vi "AnalyseLV.vi"(8 "error in (no error)":errorcluster, 10 "ImageData":T2, 11 "FluorescenceAnalyser in":refnum<class "FluorescenceAnalyser.lvclass">) -> (0 "error out":errorcluster, 3 "FluorescenceAnalyser out":refnum<class "FluorescenceAnalyser.lvclass">)   [LabVIEW 2009, in "Tools.lvlib" / "Imaging.lvlib" / "FluorescenceAnalyser.lvclass"]
uses:
  FluorescenceAnalyser.lvclass
  <vilib>/Analysis/NI_AALBase.lvlib
  ImageAnalyser.lvclass
panel:
  out "Image":T1(plugin-control)
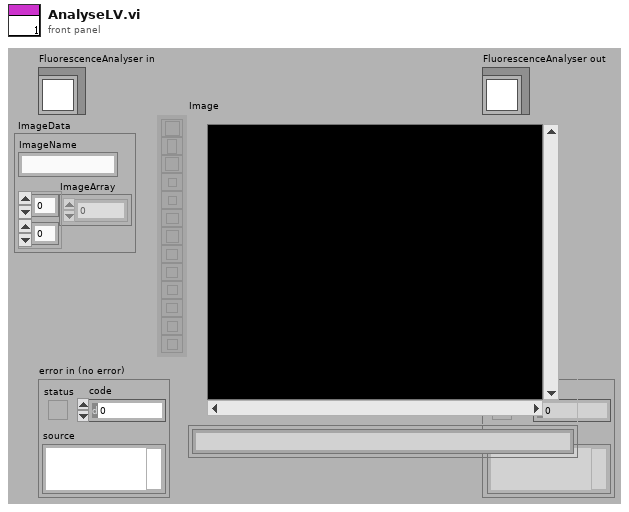
[diagram p1: front panel]
types:
  T1 = typedef "IMAQ Image.ctl" = refnum<image>
  T2 = cluster{"ImageName":string, "ImageArray":sgl[][]}
  T3 = cluster{"Name":string, "Results":dbl[], "AnalysisType":string}
  T4 = cluster{"Objects":u16, "Threshold":i32, "Reject Border":bool, "Fill Holes":bool, "Min Object Size":bool, "Min Size":i32, "Max Object Size":bool, "Max Size":i32, "Show Search Area":bool, "Show Center":bool, "Show Bounding Box":bool}
  T5 = typedef "Image Type" = u32
  T6 = cluster{"Object Center":cluster{"X":sgl, "Y":sgl}, "Bounding Box":cluster{"X Left":i32, "Y Top":i32, "X Right":i32, "Y Bottom":i32}, "Area":sgl, "Orientation":sgl, "Aspect Ratio":sgl, "Nb Holes":i32}[]
  T7 = cluster{"Object Center":cluster{"X":sgl, "Y":sgl}, "Bounding Box":cluster{"X Left":i32, "Y Top":i32, "X Right":i32, "Y Bottom":i32}, "Area":sgl, "Orientation":sgl, "Aspect Ratio":sgl, "Nb Holes":i32}
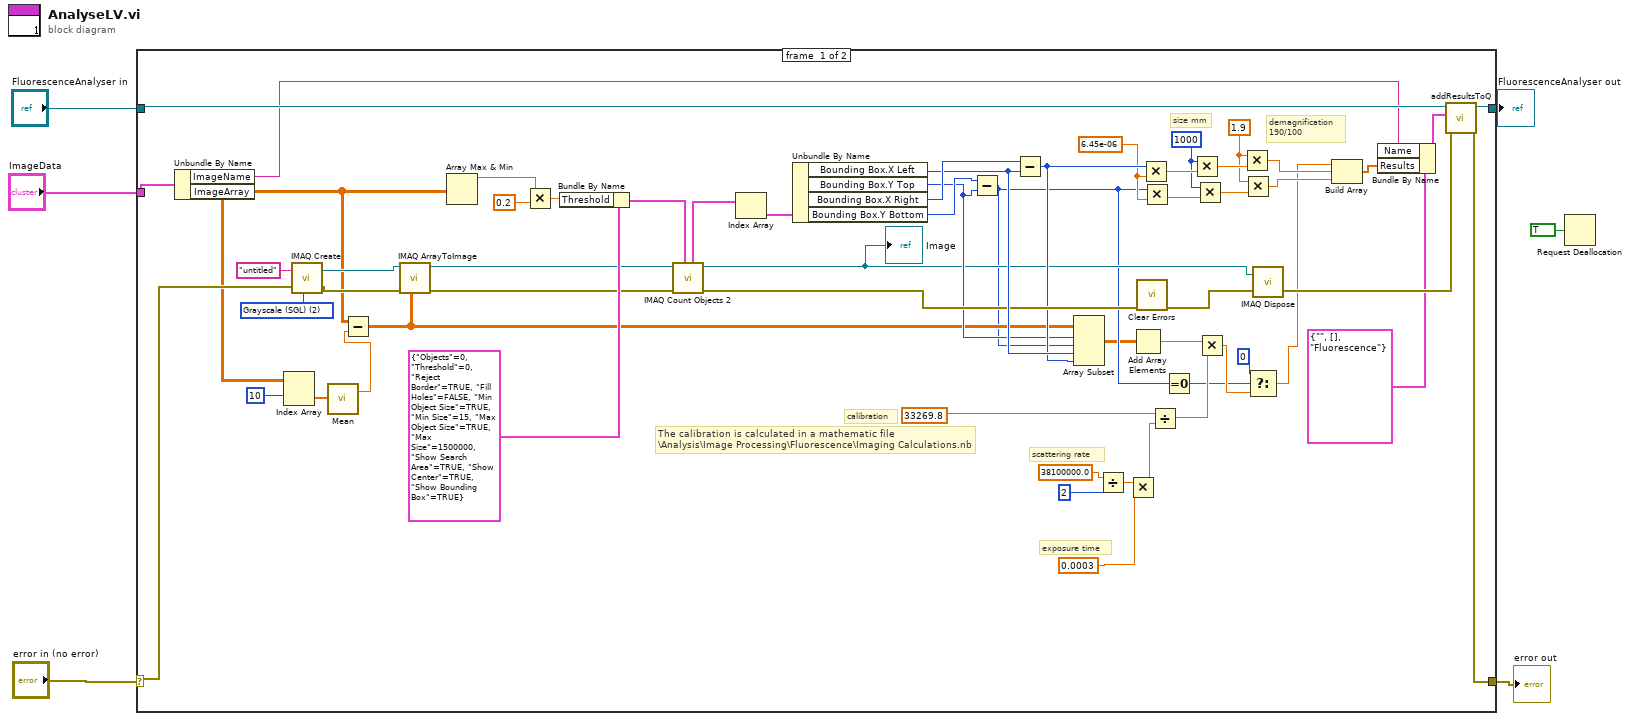
[diagram p0: block diagram]
diagram:
  n1 = case shown="No Error" "error in (no error)" {
    selector: "error in (no error)" -> [w48 w67]
    tunnel: [w33 w67] -> w5
    tunnel: [w35 w66] -> w3
    tunnel: "FluorescenceAnalyser in" -> [w34 w66]
    tunnel: "ImageData" -> [w65 _]
    frame #0 {
      w15 = 1.9
      w28 = 1000
      w46 = 6.45e-06
      w50 = T5 2 items=["Grayscale (U8)", "Grayscale (I16)", "Grayscale (SGL)", "Complex (CSG)", "RGB (U32)", "HSL (U32)", "RGB (U64)", "Grayscale (U16)"] ("Image Type")
      # "The calibration is calculated in a mathematic file\n\\Analysis\\Image Processing\\Fluorescence\\Imaging Calculations.nb"
      # "demagnification\n190/100"
      # "size mm"
      # "exposure time"
      # "scattering rate"
      # "calibration"
      n2 = Unbundle By Name(w65) -> ("ImageName"=w21:string, "ImageArray"=w24:sgl[][])
      n3 = Index Array(array=w24, index (row)=10) -> (element=w42:sgl[])  [unwired: 1 in]
      n4 = call "IMAQ Create"("Image Name"="untitled", "Image Type"=w50, "error in (no error)"=w48) -> ("New Image"=w64:T1, "error out"=w63:errorcluster)  [unwired: 2 in]
      n5 = call <vilib>:"Mean.vi"("X"=w42) -> ("mean"=w10:dbl)  [unwired: 1 out]
      n6 = Subtract(x=w24, y=w10) -> (x-y=w14:dbl[][])
      n7 = call "IMAQ ArrayToImage"("Image Pixels (Float)"=w14, "error in (no error)"=w63, "Image"=w64) -> ("error out"=w55:errorcluster, "Image Out"=w56:T1)  [unwired: 7 in]
      n8 = Array Max & Min(array=w24) -> (max value=w59:sgl)  [unwired: 3 out]
      n9 = Multiply(x=w59, y=0.2) -> (x*y=w60:dbl)
      n10 = Bundle By Name(cluster=T4 {"Objects"=0, "Threshold"=0, "Reject Border"=TRUE, "Fill Holes"=FALSE, "Min Object Size"=TRUE, "Min Size"=15, "Max Object Size"=TRUE, "Max Size"=1500000, "Show Search Area"=TRUE, "Show Center"=TRUE, "Show Bounding Box"=TRUE} ("Settings"), "Threshold"=w60) -> (w57:T4)
      n11 = call "IMAQ Count Objects 2"("Settings"=w57, "error in (no error)"=w55, "Image"=w56) -> ("error out"=w49:errorcluster, "Image Out"=w27:T1, "Objects"=w54:T6)  [unwired: 4 in, 2 out]
      "Image" <- w27
      n12 = Index Array(array=w54) -> (element=w53:T7)  [unwired: 1 in]
      n13 = Unbundle By Name(w53) -> ("Bounding Box.X Left"=w51:i32, "Bounding Box.Y Top"=w31:i32, "Bounding Box.X Right"=w52:i32, "Bounding Box.Y Bottom"=w32:i32)
      n14 = Subtract(x=w32, y=w31) -> (x-y=w9:i32)
      n15 = Subtract(x=w52, y=w51) -> (x-y=w47:i32)
      n16 = Array Subset(array=w14, index (row)=w31, length (row)=w9, index (col)=w51, length (col)=w47) -> (w7:dbl[][])
      n17 = Divide(x=38100000.0, y=2) -> (x/y=w40:dbl)
      n18 = Multiply(x=w40, y=0.0003) -> (x*y=w39:dbl)
      n19 = Add Array Elements(numeric array=w7) -> (sum=w37:dbl)
      n20 = call <vilib>:"Clear Errors.vi"("error in (no error)"=w49) -> ("error out"=w26:errorcluster)  [unwired: 6 in]
      n21 = Multiply(x=w47, y=w46) -> (x*y=w30:dbl)
      n22 = Multiply(x=w9, y=w46) -> (x*y=w29:dbl)
      n23 = Divide(x=33269.8, y=w39) -> (x/y=w36:dbl)
      n24 = Equal To 0?(x=w9) -> (x = 0?=w8:bool)
      n25 = Multiply(x=w28, y=w30) -> (x*y=w19:dbl)
      n26 = Multiply(x=w28, y=w29) -> (x*y=w18:dbl)
      n27 = Multiply(x=w37, y=w36) -> (x*y=w12:dbl)
      n28 = Multiply(x=w15, y=w19) -> (x*y=w17:dbl)
      n29 = Multiply(x=w15, y=w18) -> (x*y=w16:dbl)
      n30 = Select(t=0, s=w8, f=w12) -> (s? t:f=w11:dbl)
      n31 = call "IMAQ Dispose"("Image"=w27, "error in (no error)"=w26) -> ("error out"=w25:errorcluster)  [unwired: 4 in]
      n32 = Build Array(w11, w17, w16) -> (w22:dbl[])
      n33 = Bundle By Name(cluster=T3 {"Name"="", "Results"=[], "AnalysisType"="Fluorescence"} ("output cluster"), "Name"=w21, "Results"=w22) -> (w20:T3)
      n34 = call "addResultsToQ.vi"("error in (no error)"=w25, "Results"=w20, "ImageAnalyser in"=w34) -> ("error out"=w33:errorcluster, "ImageAnalyser out"=w35:refnum<class "FluorescenceAnalyser.lvclass">)  [unwired: 7 in]
    }
    frame #1 {
    }
  }
  "error out" <- w5
  "FluorescenceAnalyser out" <- w3
  n35 = Request Deallocation(TRUE ("flag")) -> ()
